vi "TEST.vi"   [LabVIEW 2016]
uses:
  <vilib>/Hampel Software Engineering/HSE Logger/LogLevel.ctl
  <vilib>/Hampel Software Engineering/HSE Logger/Handler/FileHandler/FileHandler.lvclass
  C:/Program Files (x86)/National Instruments/LabVIEW 2016/vi.lib/Hampel Software Engineering/HSE Logger/Handler/Handler.lvclass
  <vilib>/Hampel Software Engineering/HSE Logger/hse-logger.lvlib
types:
  T1 = typedef "hse-logger.lvlib/LogLevel.ctl" = enum16{"DEBUG", "INFO", "WARNING", "ERROR", "CRITICAL"}
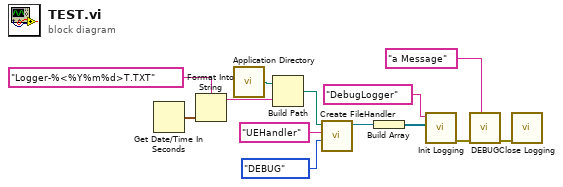
[diagram p0: block diagram]
diagram:
  n1 = Get Date/Time In Seconds() -> (seconds since 1Jan1904=w3:timestamp)
  n2 = Format Into String(format string="Logger-%<%Y%m%d>T.TXT", w3) -> (resulting string=w4:string)  [unwired: 2 in, 1 out]
  n3 = call <vilib>:"Application Directory.vi"() -> ("Application Directory"=w6:path)
  n4 = Build Path(base path=w6, name or relative path=w4) -> (appended path=w5:path)
  n5 = call <vilib>:"Create FileHandler.vi"("Level"=LogLevel."DEBUG", "Name"="UEHandler", "Filepath"=w5) -> ("FileHandler out"=w8:refnum<class "FileHandler.lvclass">)  [unwired: 7 in, 1 out]
  n6 = Build Array(w8) -> (w11:refnum<class "FileHandler.lvclass">[])
  n7 = call <vilib>:"Init Logging.vi"("Handlers"=w11, "Name"="DebugLogger") -> ("error out"=w9:errorcluster)  [unwired: 9 in]
  n8 = call <vilib>:"DEBUG.vi"("Message"="a Message", "error in"=w9) -> ("error out"=w10:errorcluster)  [unwired: 9 in]
  n9 = call <vilib>:"Close Logging.vi"("error in"=w10) -> ()  [unwired: 10 in, 1 out]
